vi "MAIN - Template Application.vi"() -> ()   [LabVIEW 2012, in "Car Wash.lvlib"]
uses:
  Car Wash.lvlib
  Components/State Declaration.ctl
  Components/System Trigger.ctl
  Components/System Trigger Element.ctl
  <vilib>/Utility/error.llb/DialogTypeEnum.ctl
  Components/AMC/Read Termination Message.vi
  Components/AMC/Update Message Routing Info.vi
  Components/AMC/Create Multiple Messages.vi
  Components/AMC/Create Single Message.vi
  Components/TypeDef - SHIFTER.ctl
  Components/AMC/Globals.vi
  Components/AMC/Send Message.vi
  Components/Dependencies.llb/TLB`_Dependencies.lvlib
  Components/AMC/AMC.lvlib
panel:
  out "Status":string
  in  "Start Wash":bool
  in  "Reset Car":bool
  out "Wash Progress":dbl(slide) scale=0.0..6.0
  in  "Giant Blowdryers":bool
  in  "Rinse":bool
  in  "Wax":bool
  in  "Roller Brushes":bool
  in  "Soap":bool
  in  "Pre-Soak":bool
  out "error out":errorcluster
  # "Car Wash"
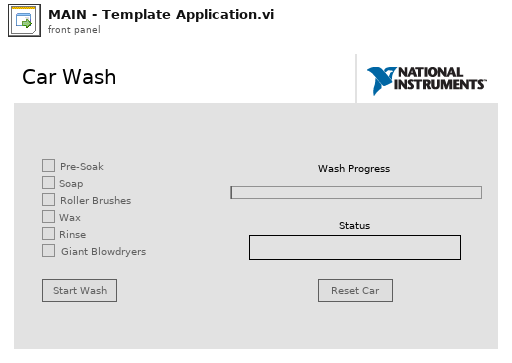
[diagram p1: front panel]
types:
  T1 = typedef "Car Wash.lvlib/System Trigger.ctl" = enum16{"<None>", "Cache User Parameters", "Close Application", "Start Wash", "Reset Car"}
  T2 = typedef "Car Wash.lvlib/State Declaration.ctl" = enum16{"<Startup>", "Idle", "Washing", "Done Washing", "<Shutdown>"}
  T3 = enum16{"Clear SR", "Set Display", "Set Shifter", "Initialize Events", "Init Q"}
  T4 = typedef "Car Wash.lvlib/TypeDef - SHIFTER.ctl" = cluster{"State":T2, "User Data":cluster{"Active Item Tag":string, "Pre-Soak":bool, "Soap":bool, "Roller Brushes":bool, "Wax":bool, "Rinse":bool, "Giant Blowdryers":bool}, "Display Data":cluster{"Active Item Tag":string, "Wash Progress":dbl, "Status":string}, "User Parameter Controls":refnum<vi>[], "Framework Data":cluster{"Exit Event":T5, "Terminate Error":errorcluster}, "Private Data":cluster{"Active Item Tag":string, "Step Booleans Array":bool[], "Step Names Array":string[]}}
  T5 = typedef "Car Wash.lvlib/TLB`_Dependencies.lvlib/Exit Event Ref.ctl" = refnum<user-event>
  T6 = typedef "Car Wash.lvlib/System Trigger Element.ctl" = cluster{"System Triggers":T1, "Trigger Data":variant}
  T7 = typedef "Car Wash.lvlib/AMC.lvlib/Message Queue.ctl" = refnum<queue>
  T8 = enum8{"Enabled", "Disabled", "Disabled and Grayed Out"}
  T9 = typedef "DialogTypeEnum.ctl" = enum16{"no dialog", "OK message", "continue or stop message", "auto error handling dialog", "OK message + warnings", "continue/stop + warnings"}
  T10 = enum32{"Invalid", "Standard", "Closed", "Hidden", "Minimized", "Maximized"}
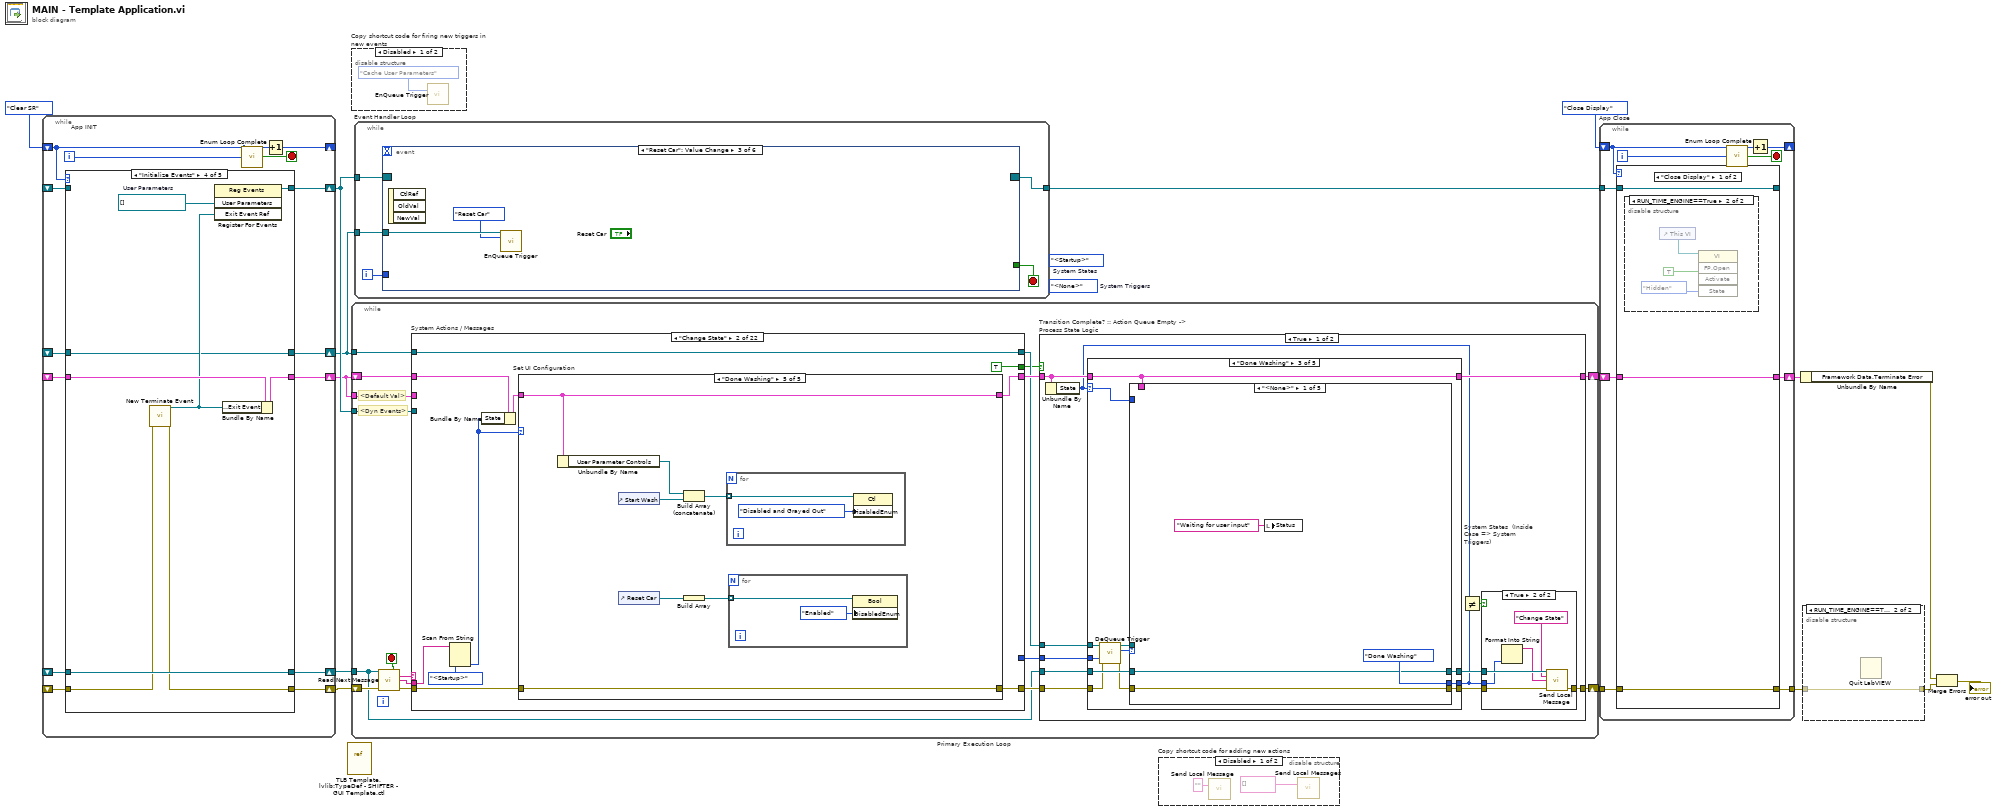
[diagram p0: block diagram]
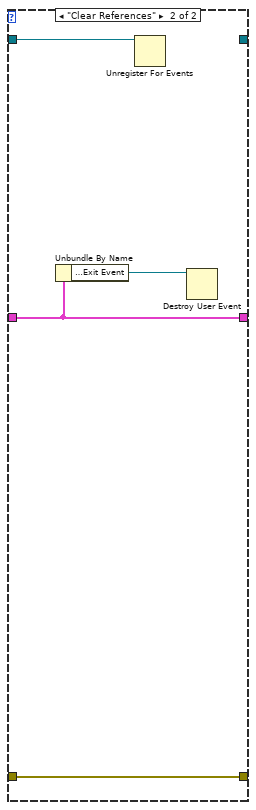
[diagram p6: hidden frame]
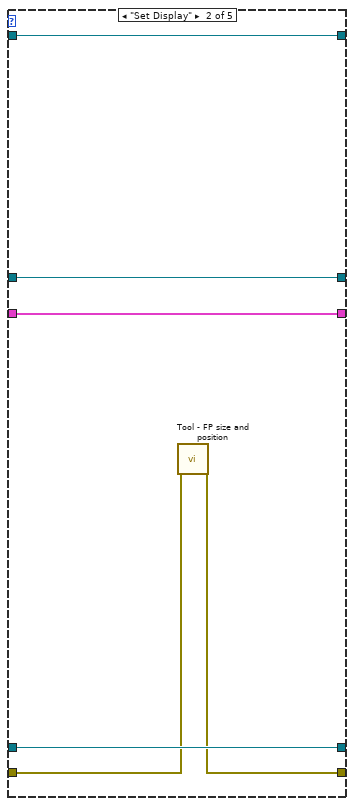
[diagram p8: hidden frame]
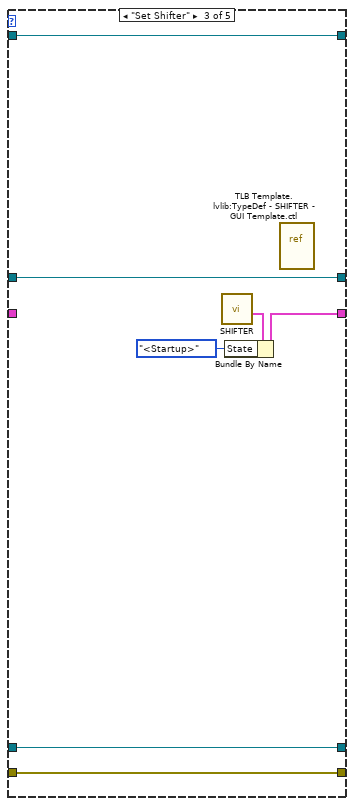
[diagram p9: hidden frame]
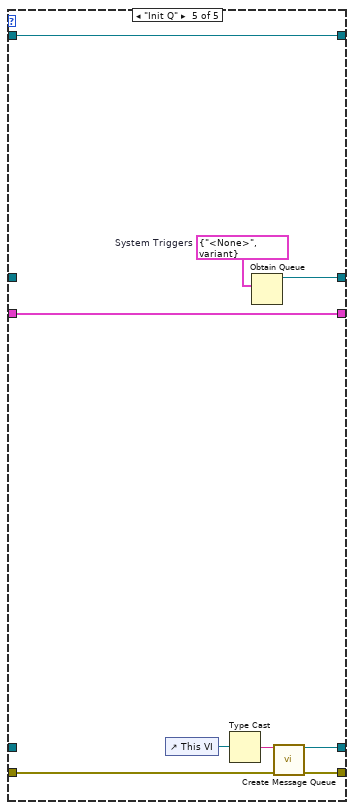
[diagram p10: hidden frame]
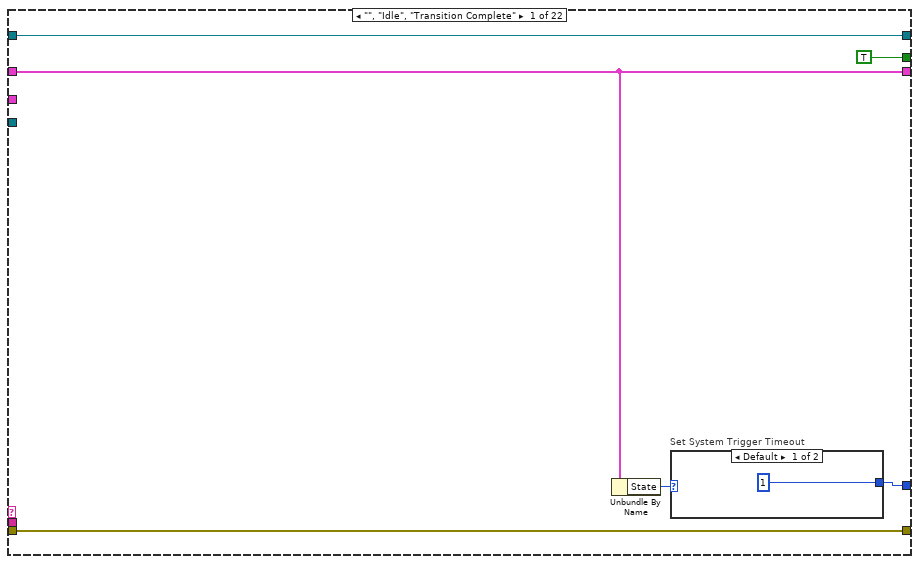
[diagram p11: hidden frame]
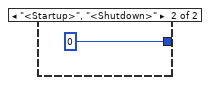
[diagram p12: hidden frame]
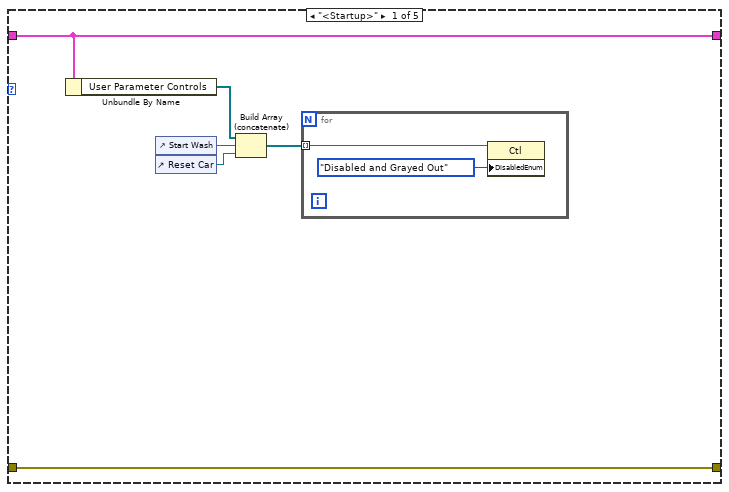
[diagram p13: hidden frame]
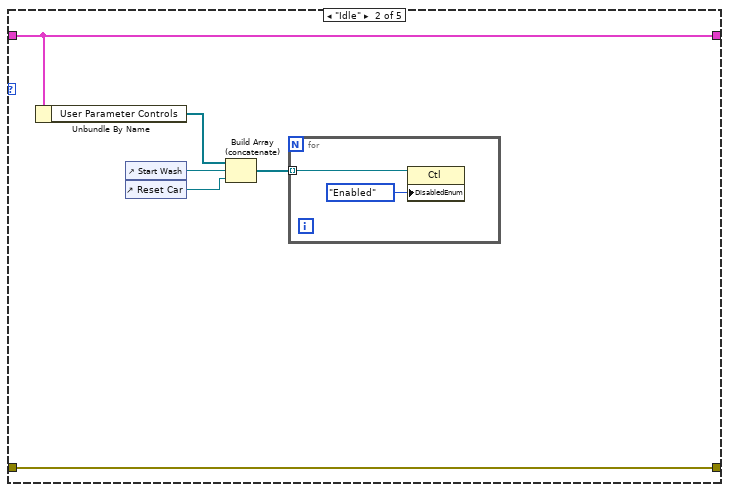
[diagram p14: hidden frame]
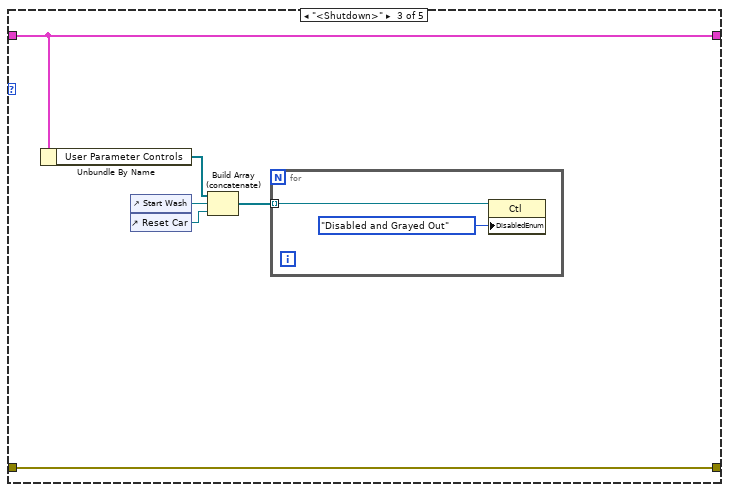
[diagram p15: hidden frame]
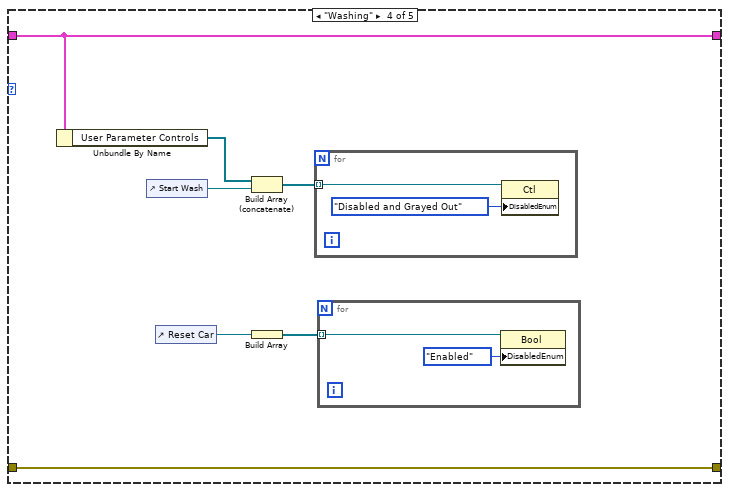
[diagram p16: hidden frame]
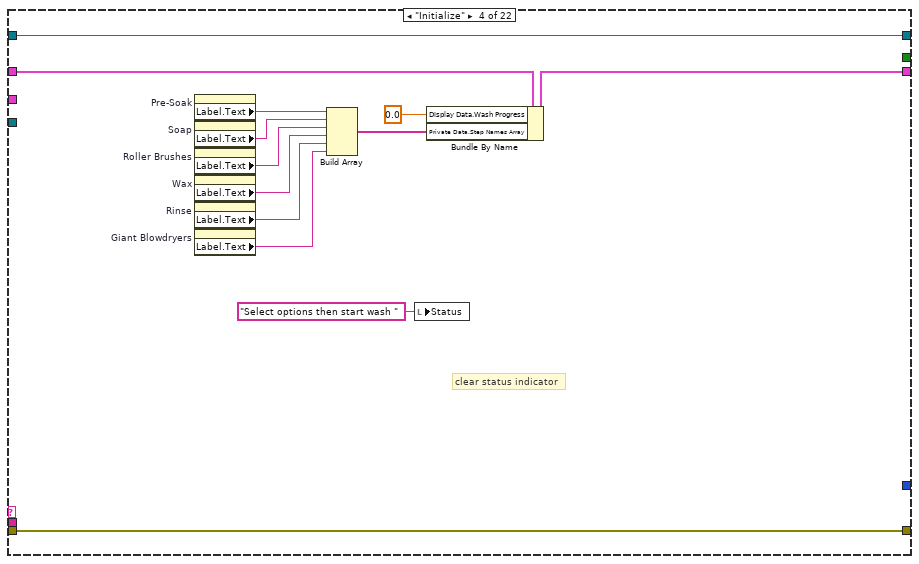
[diagram p18: hidden frame]
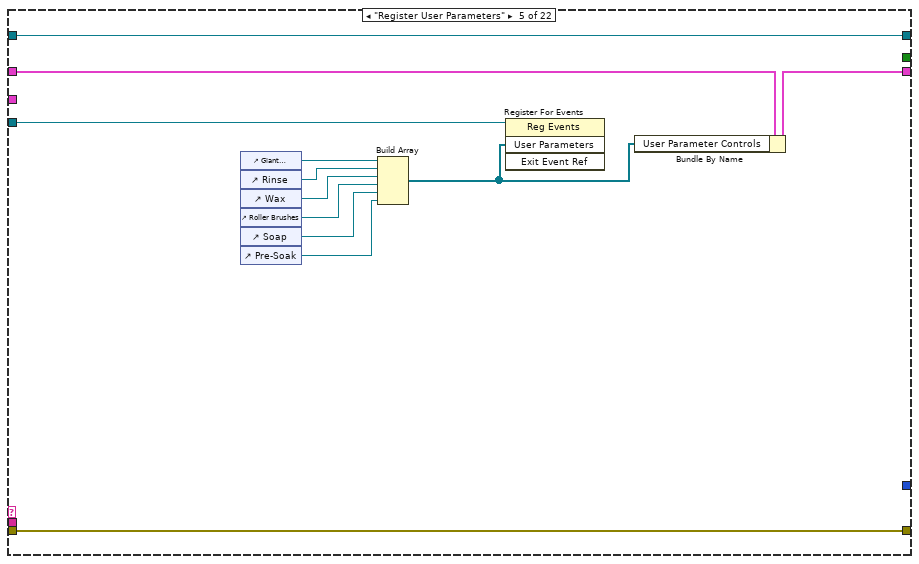
[diagram p19: hidden frame]
diagram:
  (unwired) System_Trigger."<None>"  # System Triggers
  (unwired) State_Declaration."<Startup>"  # System States
  n1 = while "App INIT" {
    shift-right: [w23] -> _
    shift-left: T3."Clear SR" -> [w18]
    shift-right: [w29] -> w9
    shift-left: _ -> [w22]
    shift-right: [w26] -> w8
    shift-left: _ -> [w21]
    shift-right: [w28] -> w11
    shift-left: _ -> [w20]
    shift-right: [w27] -> w1
    shift-left: _ -> [w19]
    shift-right: [w17] -> w2
    shift-left: _ -> [w16]
    i -> [w24]
    stop <- w25 stop-if-true
    n2 = case shown="\"Initialize Events\"" w18 {
      tunnel: [_ w33 w42 w51 w56] -> w29
      tunnel: [_ w31 w41 w44 w55] -> w26
      tunnel: [_ w35 w36 w48 w54] -> w27
      tunnel: [_ w34 w40 w47 w60] -> w28
      tunnel: w22 -> [_ w33 w42 w51 _]
      tunnel: w21 -> [_ w32 w41 w45 w59]
      tunnel: w20 -> [_ w34 w40 _ w60]
      tunnel: w19 -> [_ w35 _ w49 w54]
      tunnel: [_ w30 w39 w43 w58] -> w17
      tunnel: w16 -> [_ w30 w39 w43 _]
      frame "Clear SR" {
      }
      frame "Set Display" {
        n3 = call "Tool - FP size and position.vi"("error in (no error)"=w32) -> ("error out"=w31:errorcluster)  [unwired: 7 in, 11 out]
      }
      frame "Set Shifter" {
        n4 = call "SHIFTER.vi"() -> ("SHIFTER DATA"=w37:T4)  [unwired: 15 in]
        n5 = Bundle By Name(cluster=w37, "State"=State_Declaration."<Startup>") -> (w36:T4)
        n6 = vi-ref "TLB Template.lvlib:TypeDef - SHIFTER - GUI Template.ctl"() -> ()  [unwired: 1 out]
      }
      frame "Initialize Events" {
        w50 = refnum<vi>[] []  # User Parameters
        n7 = call "New Terminate Event.vi"("error in (no error)"=w45) -> ("Exit Event Ref"=w46:T5, "error out"=w44:errorcluster)  [unwired: 13 in]
        n8 = register-events(w50, w46) -> (reference out=w47:refnum<event-registration>)  [unwired: 2 in, 1 out]
        n9 = Bundle By Name(cluster=w49, "Framework Data.Exit Event"=w46) -> (w48:T4)
      }
      frame "Init Q" {
        w57 = T6 {"System Triggers"=enum."<None>", "Trigger Data"=variant}  # System Triggers
        n10 = control-ref of="This VI"() -> (w53:refnum<vi>)
        n11 = Type Cast(x=w53) -> (*(type *) &x=w52:string)  [unwired: 1 in]
        n12 = Obtain Queue(element data type=w57) -> (queue out=w58:refnum<queue>)  [unwired: 4 in, 2 out]
        n13 = call "Create Message Queue.vi"("message queue name"=w52, "error in"=w59) -> ("message queue out"=w56:T7, "error out"=w55:errorcluster)  [unwired: 12 in]
      }
    }
    n14 = call "Enum Loop Complete.vi"("Current State Enum"=w18, "Itteration"=w24) -> ("Loop Complete?"=w25:bool)  [unwired: 13 out]
    n15 = Increment(x=w18) -> (x+1=w23:T3)
  }
  n16 = vi-ref "TLB Template.lvlib:TypeDef - SHIFTER - GUI Template.ctl"() -> ()  [unwired: 1 out]
  n17 = disable-structure "Copy shortcut code for firing new triggers in new events" shown="Disabled" {
    frame Disabled {
      n18 = call "EnQueue Trigger.vi"("System Triggers"=System_Trigger."Cache User Parameters") -> ()  [unwired: 13 in, 2 out]
    }
    frame Enabled {
    }
  }
  n19 = while "Primary Execution Loop" {
    shift-right: [w68] -> w15
    shift-left: w8 -> [w75]
    shift-right: [w71] -> w14
    shift-left: w1 -> [w78]
    tunnel: w1 -> [w77]
    tunnel: w9 -> [w66]
    tunnel: w11 -> [w76]
    tunnel: w2 -> [w67]
    stop <- w73 stop-if-true
    # "<Dyn Events>"
    # "<Default Val>"
    n20 = call "Read Next Message.vi"("message queue in"=w66, "error in"=w75) -> ("exit process?"=w73:bool, "message name"=w72:string, "message value"=w63:string, "error out"=w74:errorcluster)  [unwired: 6 in, 4 out]
    n21 = case "System Actions / Messages" shown="\"Change State\"" w72 {
      selector: w72 -> [_ _ _ _ _ _ _ _ _ _ _ _ _ _ _ _ _ _ _ _ _ w326]
      tunnel: [w84 w91 w145 w157 w170 w173 w181 w187 w190 w201 w207 w215 w224 w236 w248 w260 w272 w284 w292 w297 w320 w330] -> w69
      tunnel: w74 -> [w84 w90 w145 w157 w170 w173 w181 w187 w190 w201 w207 w215 w224 w236 w248 w260 w272 w284 w292 w298 w319 w331]
      tunnel: w78 -> [w79 w87 w144 w156 w169 w172 w183 w185 w188 w193 w204 w213 w220 w232 w244 w256 w268 w280 w291 w295 w323 w332]
      tunnel: w77 -> [_ _ _ _ _ _ _ _ _ _ _ _ _ _ _ _ _ _ _ _ _ _]
      tunnel: [w79 w89 w144 w155 w168 w172 w182 w185 w188 w192 w203 w213 w219 w231 w243 w255 w267 w279 w291 w296 w323 w332] -> w70
      tunnel: [w80 _ _ _ _ _ _ _ _ _ _ _ _ _ _ _ _ _ _ _ _ _] -> w62
      tunnel: w76 -> [_ _ _ _ w167 _ _ _ _ _ _ _ _ _ _ _ _ _ _ _ _ _]
      tunnel: [w82 w95 w143 w158 w166 w171 w180 w186 w189 w200 w206 w214 w223 w235 w247 w259 w271 w283 w290 w293 w317 w324] -> w65
      tunnel: w67 -> [w82 w95 w143 w158 w166 w171 w180 w186 w189 w200 w206 w214 w223 w235 w247 w259 w271 w283 w290 w293 w317 w324]
      tunnel: [TRUE TRUE _ _ _ _ _ _ _ _ _ _ _ _ _ _ _ _ _ _ _ _] -> w64
      tunnel: w63 -> [_ w94 _ _ _ _ _ _ _ _ _ _ _ _ _ _ _ _ _ _ _ _]
      frame "", "Idle", "Transition Complete" {
        n22 = Unbundle By Name(w79) -> ("State"=w81:T2)
        n23 = case "Set System Trigger Timeout" shown="Default" w81 {
          tunnel: [1 0] -> w80
          frame Default {
          }
          frame "<Startup>", "<Shutdown>" {
          }
        }
      }
      frame "Change State" {
        n24 = Scan From String(input string=w94, default 1=State_Declaration."<Startup>" ("State")) -> (output 1=w92:T2)  [unwired: 3 in, 3 out]
        n25 = Bundle By Name(cluster=w87, "State"=w92) -> (w88:T4)
        n26 = case "Set UI Configuration" shown="\"Done Washing\"" w92 {
          tunnel: [w102 w110 w118 w127 w138] -> w91
          tunnel: w90 -> [w102 w110 w118 w127 w138]
          tunnel: [w98 w106 w114 w122 w133] -> w89
          tunnel: w88 -> [w98 w106 w114 w122 w133]
          frame "<Startup>" {
            n27 = Unbundle By Name(w98) -> ("User Parameter Controls"=w97:refnum<vi>[])
            n28 = control-ref of="Start Wash"() -> (w101:refnum<vi>)
            n29 = control-ref of="Reset Car"() -> (w99:refnum<vi>)
            n30 = Build Array (concatenate)(w97, w101, w99) -> (w100:refnum<vi>[])
            n31 = for {
              tunnel: w100 -> [w104] mode=indexing
              n32 = property class="Ctl"(reference=w104, "DisabledEnum"=T8."Disabled and Grayed Out" ("Disabled")) -> ()  [unwired: 1 in, 2 out]
            }
          }
          frame "Idle" {
            n33 = Unbundle By Name(w106) -> ("User Parameter Controls"=w105:refnum<vi>[])
            n34 = control-ref of="Start Wash"() -> (w108:refnum<vi>)
            n35 = control-ref of="Reset Car"() -> (w107:refnum<vi>)
            n36 = Build Array (concatenate)(w105, w108, w107) -> (w109:refnum<vi>[])
            n37 = for {
              tunnel: w109 -> [w112] mode=indexing
              n38 = property class="Ctl"(reference=w112, "DisabledEnum"=T8."Enabled" ("Disabled")) -> ()  [unwired: 1 in, 2 out]
            }
          }
          frame "<Shutdown>" {
            n39 = Unbundle By Name(w114) -> ("User Parameter Controls"=w113:refnum<vi>[])
            n40 = control-ref of="Start Wash"() -> (w116:refnum<vi>)
            n41 = control-ref of="Reset Car"() -> (w115:refnum<vi>)
            n42 = Build Array (concatenate)(w113, w116, w115) -> (w117:refnum<vi>[])
            n43 = for {
              tunnel: w117 -> [w120] mode=indexing
              n44 = property class="Ctl"(reference=w120, "DisabledEnum"=T8."Disabled and Grayed Out" ("Disabled")) -> ()  [unwired: 1 in, 2 out]
            }
          }
          frame "Washing" {
            n45 = Unbundle By Name(w122) -> ("User Parameter Controls"=w121:refnum<vi>[])
            n46 = control-ref of="Start Wash"() -> (w125:refnum<vi>)
            n47 = control-ref of="Reset Car"() -> (w123:refnum<vi>)
            n48 = Build Array (concatenate)(w121, w125) -> (w126:refnum<vi>[])
            n49 = Build Array(w123) -> (w124:refnum<vi>[])
            n50 = for {
              tunnel: w126 -> [w131] mode=indexing
              n51 = property class="Ctl"(reference=w131, "DisabledEnum"=T8."Disabled and Grayed Out" ("Disabled")) -> ()  [unwired: 1 in, 2 out]
            }
            n52 = for {
              tunnel: w124 -> [w129] mode=indexing
              n53 = property class="Bool"(reference=w129, "DisabledEnum"=T8."Enabled" ("Disabled")) -> ()  [unwired: 1 in, 2 out]
            }
          }
          frame "Done Washing" {
            n54 = Unbundle By Name(w133) -> ("User Parameter Controls"=w132:refnum<vi>[])
            n55 = control-ref of="Start Wash"() -> (w136:refnum<vi>)
            n56 = control-ref of="Reset Car"() -> (w134:refnum<vi>)
            n57 = Build Array (concatenate)(w132, w136) -> (w137:refnum<vi>[])
            n58 = Build Array(w134) -> (w135:refnum<vi>[])
            n59 = for {
              tunnel: w137 -> [w142] mode=indexing
              n60 = property class="Ctl"(reference=w142, "DisabledEnum"=T8."Disabled and Grayed Out" ("Disabled")) -> ()  [unwired: 1 in, 2 out]
            }
            n61 = for {
              tunnel: w135 -> [w140] mode=indexing
              n62 = property class="Bool"(reference=w140, "DisabledEnum"=T8."Enabled" ("Disabled")) -> ()  [unwired: 1 in, 2 out]
            }
          }
        }
      }
      frame "/*********Initialize********/" {
      }
      frame "Initialize" {
        # "clear status indicator"
        n63 = property on="Pre-Soak" class="Bool (strict)"() -> ("Label.Text"=w152:string)  [unwired: 2 in, 2 out]
        n64 = property on="Soap" class="Bool (strict)"() -> ("Label.Text"=w151:string)  [unwired: 2 in, 2 out]
        n65 = property on="Roller Brushes" class="Bool (strict)"() -> ("Label.Text"=w150:string)  [unwired: 2 in, 2 out]
        n66 = property on="Wax" class="Bool (strict)"() -> ("Label.Text"=w149:string)  [unwired: 2 in, 2 out]
        n67 = property on="Rinse" class="Bool (strict)"() -> ("Label.Text"=w148:string)  [unwired: 2 in, 2 out]
        n68 = property on="Giant Blowdryers" class="Bool (strict)"() -> ("Label.Text"=w147:string)  [unwired: 2 in, 2 out]
        n69 = Build Array(w152, w151, w150, w149, w148, w147) -> (w146:string[])
        n70 = local write "Status"("Select options then start wash " ("Status")) -> ()
        n71 = Bundle By Name(cluster=w156, "Display Data.Wash Progress"=0.0, "Private Data.Step Names Array"=w146) -> (w155:T4)
      }
      frame "Register User Parameters" {
        n72 = control-ref of="Giant Blowdryers"() -> (w165:refnum<vi>)
        n73 = control-ref of="Rinse"() -> (w160:refnum<vi>)
        n74 = control-ref of="Wax"() -> (w161:refnum<vi>)
        n75 = control-ref of="Roller Brushes"() -> (w162:refnum<vi>)
        n76 = control-ref of="Soap"() -> (w163:refnum<vi>)
        n77 = control-ref of="Pre-Soak"() -> (w164:refnum<vi>)
        n78 = Build Array(w165, w160, w161, w162, w163, w164) -> (w159:refnum<vi>[])
        n79 = register-events(reference=w167, w159) -> ()  [unwired: 2 in, 2 out]
        n80 = Bundle By Name(cluster=w169, "User Parameter Controls"=w159) -> (w168:T4)
      }
      frame "/*********Display Updates********/" {
      }
      frame "Cache User Parameters" {
        n81 = Bundle By Name(cluster=w183, "User Data.Pre-Soak"="Pre-Soak", "User Data.Soap"="Soap", "User Data.Roller Brushes"="Roller Brushes", "User Data.Wax"="Wax", "User Data.Rinse"="Rinse", "User Data.Giant Blowdryers"="Giant Blowdryers") -> (w182:T4)
      }
      frame "Update Display" {
        # "status updated via local variable"
        n82 = Unbundle By Name(w185) -> ("Display Data.Wash Progress"=→"Wash Progress":dbl)
      }
      frame "/*********Primary Execution********/" {
      }
      frame "Create Steps Array" {
        n83 = Unbundle By Name(w193) -> ("User Data.Pre-Soak"=w199:bool, "User Data.Soap"=w198:bool, "User Data.Roller Brushes"=w197:bool, "User Data.Wax"=w196:bool, "User Data.Rinse"=w195:bool, "User Data.Giant Blowdryers"=w194:bool)
        n84 = Build Array(w199, w198, w197, w196, w195, w194) -> (w191:bool[])
        n85 = Bundle By Name(cluster=w193, "Private Data.Step Booleans Array"=w191) -> (w192:T4)
      }
      frame "Increment Step" {
        n86 = Unbundle By Name(w204) -> ("Display Data.Wash Progress"=w205:dbl)
        n87 = Increment(x=w205) -> (x+1=w202:dbl)
        n88 = Bundle By Name(cluster=w204, "Display Data.Wash Progress"=w202) -> (w203:T4)
      }
      frame "Evaluate Step" {
        n89 = Unbundle By Name(w213) -> ("Display Data.Wash Progress"=w210:dbl, "Private Data.Step Booleans Array"=w212:bool[], "Private Data.Step Names Array"=w211:string[])
        n90 = Index Array(array=w211, index=w210) -> (element=w208:string)
        n91 = Index Array(array=w212, index=w210) -> (element=w209:bool)
        n92 = case shown="True" w209 {
          tunnel: w208 -> [_ w217]
          frame False {
          }
          frame True {
            n93 = local write "Status"(w217) -> ()
            n94 = Wait (ms)(milliseconds to wait=u32 1000 ("millisecond timer value")) -> ()  [unwired: 1 out]
          }
        }
      }
      frame "Pre-Soak" {
        n95 = Unbundle By Name(w220) -> ("Display Data.Wash Progress"=w222:dbl)
        n96 = Unbundle By Name(w220) -> ("User Data.Pre-Soak"=w218:bool)
        n97 = case shown="True" w218 {
          tunnel: w222 -> [w225 w229]
          tunnel: [w225 w228] -> w221
          frame False {
          }
          frame True {
            n98 = Increment(x=w229) -> (x+1=w228:dbl)
            n99 = local write "Status"("Pre-Soak" ("Status")) -> ()
            n100 = Wait (ms)(milliseconds to wait=u32 1000) -> ()  [unwired: 1 out]
          }
        }
        n101 = Bundle By Name(cluster=w220, "Display Data.Wash Progress"=w221) -> (w219:T4)
      }
      frame "Soap" {
        n102 = Unbundle By Name(w232) -> ("Display Data.Wash Progress"=w234:dbl)
        n103 = Unbundle By Name(w232) -> ("User Data.Soap"=w230:bool)
        n104 = case shown="True" w230 {
          tunnel: w234 -> [w237 w241]
          tunnel: [w237 w240] -> w233
          frame False {
          }
          frame True {
            n105 = Increment(x=w241) -> (x+1=w240:dbl)
            n106 = local write "Status"("Soap" ("Status")) -> ()
            n107 = Wait (ms)(milliseconds to wait=u32 1000) -> ()  [unwired: 1 out]
          }
        }
        n108 = Bundle By Name(cluster=w232, "Display Data.Wash Progress"=w233) -> (w231:T4)
      }
      frame "Roller Brushes" {
        n109 = Unbundle By Name(w244) -> ("Display Data.Wash Progress"=w246:dbl)
        n110 = Unbundle By Name(w244) -> ("User Data.Roller Brushes"=w242:bool)
        n111 = case shown="True" w242 {
          tunnel: w246 -> [w249 w253]
          tunnel: [w249 w252] -> w245
          frame False {
          }
          frame True {
            n112 = Increment(x=w253) -> (x+1=w252:dbl)
            n113 = local write "Status"("Roller Brushes" ("Status")) -> ()
            n114 = Wait (ms)(milliseconds to wait=u32 1000) -> ()  [unwired: 1 out]
          }
        }
        n115 = Bundle By Name(cluster=w244, "Display Data.Wash Progress"=w245) -> (w243:T4)
      }
      frame "Wax" {
        n116 = Unbundle By Name(w256) -> ("Display Data.Wash Progress"=w258:dbl)
        n117 = Unbundle By Name(w256) -> ("User Data.Wax"=w254:bool)
        n118 = case shown="True" w254 {
          tunnel: w258 -> [w261 w265]
          tunnel: [w261 w264] -> w257
          frame False {
          }
          frame True {
            n119 = Increment(x=w265) -> (x+1=w264:dbl)
            n120 = local write "Status"("Wax" ("Status")) -> ()
            n121 = Wait (ms)(milliseconds to wait=u32 1000) -> ()  [unwired: 1 out]
          }
        }
        n122 = Bundle By Name(cluster=w256, "Display Data.Wash Progress"=w257) -> (w255:T4)
      }
      frame "Rinse" {
        n123 = Unbundle By Name(w268) -> ("Display Data.Wash Progress"=w270:dbl)
        n124 = Unbundle By Name(w268) -> ("User Data.Rinse"=w266:bool)
        n125 = case shown="True" w266 {
          tunnel: w270 -> [w273 w277]
          tunnel: [w273 w276] -> w269
          frame False {
          }
          frame True {
            n126 = Increment(x=w277) -> (x+1=w276:dbl)
            n127 = local write "Status"("Rinse" ("Status")) -> ()
            n128 = Wait (ms)(milliseconds to wait=u32 1000) -> ()  [unwired: 1 out]
          }
        }
        n129 = Bundle By Name(cluster=w268, "Display Data.Wash Progress"=w269) -> (w267:T4)
      }
      frame "Giant Blowdryers" {
        n130 = Unbundle By Name(w280) -> ("Display Data.Wash Progress"=w282:dbl)
        n131 = Unbundle By Name(w280) -> ("User Data.Giant Blowdryers"=w278:bool)
        n132 = case shown="True" w278 {
          tunnel: w282 -> [w285 w289]
          tunnel: [w285 w288] -> w281
          frame False {
          }
          frame True {
            n133 = Increment(x=w289) -> (x+1=w288:dbl)
            n134 = local write "Status"("Giant Blowdryers" ("Status")) -> ()
            n135 = Wait (ms)(milliseconds to wait=u32 1000) -> ()  [unwired: 1 out]
          }
        }
        n136 = Bundle By Name(cluster=w280, "Display Data.Wash Progress"=w281) -> (w279:T4)
      }
      frame "/*********Shutdown********/" {
      }
      frame "Error" {
        n137 = Unbundle By Name(w295) -> ("State"=w294:T2)
        n138 = case shown="Default" w294 {
          tunnel: w298 -> [w306]
          tunnel: [w305] -> w297
          tunnel: w295 -> [w302]
          tunnel: [w301] -> w296
          tunnel: w293 -> [w299]
          frame Default {
            n139 = call <vilib>:"General Error Handler CORE.vi"("type of dialog (OK msg:1)"=DialogTypeEnum."auto error handling dialog", "error in (no error)"=w306) -> ("stop event propagated"=w304:bool, "error out"=w300:errorcluster)  [unwired: 12 out]
            n140 = case "User Chose to Stop and Not Continue\nFALSE = Continue: CLEAR ERRORS" shown="False" w304 {
              tunnel: [w307 w312] -> w305
              tunnel: w300 -> [w308 w314]
              tunnel: w302 -> [w309 w316]
              tunnel: [w309 w315] -> w301
              tunnel: w299 -> [_ w313]
              frame False {
                n141 = call <vilib>:"Clear Errors.vi"("error in (no error)"=w308) -> ("error out"=w307:errorcluster)  [unwired: 6 out]
              }
              frame True {
                n142 = call <vilib>:"Clear Errors.vi"("error in (no error)"=w314) -> ("error out"=w311:errorcluster)  [unwired: 6 out]
                n143 = Bundle By Name(cluster=w316, "Framework Data.Terminate Error"=w314) -> (w315:T4)
                n144 = call "EnQueue Trigger.vi"("Queue in"=w313, "System Triggers"=System_Trigger."Close Application", "error in (no error)"=w311) -> ("error out"=w312:errorcluster)  [unwired: 11 in, 1 out]
              }
            }
          }
        }
      }
      frame "Exit" {
        w318 = refnum<class> refnum  # event data
        # "Don't wire 'Error In'\nMust Execute Regardless"
        n145 = Unbundle By Name(w323) -> ("Framework Data.Exit Event"=w322:T5)  [unwired: 1 out]
        n146 = Generate User Event(user event=w322, event data cluster=w318) -> (error out=w321:errorcluster)  [unwired: 1 in, 1 out]
        n147 = Merge Errors(w321, w319) -> (w320:errorcluster)
      }
      frame Default {
        w328 = 1 items=["No error", "Argument error", "Memory is full", "Out of zone", "End of file", "File already open", "Generic file I/O error", "File not found", "File permission error", "Disk is full", "Duplicate path", "Too many files open", "System feature not enabled", "Resource file not found", "Cannot add resource", "Resource not found", "Image not found", "Image memory error", "Pen does not exist", "Config type invalid", "Config token not found", "Config parse error", "Config memory error", "Bad external code format", "Bad external code offset", "External code not present", "Null window", "Destroy window error", "Null menu", "Print aborted", "Bad print record", "Print driver error", "Windows error during printing", "Memory error during printing", "Print dialog error", "Generic print error", "Invalid device refnum", "Device not found", "Device parameter error", "Device unit error", "Cannot open device", "Device call aborted", "Generic error", "Cancelled by user", "Object ID too low", "Object ID too high", "Object not in heap", "Unknown heap", "Unknown object (invalid DefProc)", "Unknown object (DefProc not in table)", "Message out of range", "Invalid (null) method", "Unknown message", "Manager call not supported", "Bad address", "Network operation in progress", "Network operation timed out", "Connection is busy", "Network attribute not supported", "Network error", "Address in use", "System out of memory", "Connection aborted", "Connection refused", "Not connected", "Already connected", "Connection closed", "Initialization error (interapplication manager)", "Bad occurrence", "Wait on unbound occurrence handler", "Occurrence queue overflow", "Datalog type conflict", "Unused", "Unrecognized type (interapplication manager)", "Memory corrupt", "Failed to make temporary DLL", "Old CIN version", "Drag socket not found", "Failed to load drop-object", "Failed to register OLE object", "Failed to release OLE object", "Format specifier type mismatch", "Unknown format specifier", "Too few format specifiers", "Too many format specifiers", "Scan failed", "Newer CIN version", "Error converting to variant", "Runtime menu error", "Password tampered", "Variant attribute not found", "Incompatible variant data type", "Event data is not available", "Event Store is not present", "Occurrence is not found", "Event Queue is not created", "Event info is not available", "Refnum passed is NULL", "Error retrieving Class GUID", "Error retrieving CoClass GUID", "Error retrieving TypeLib GUID.", "Bad built application magic bytes.", "Specific driver is different from the specific driver associated with the Logical Name.", "There is no session opened to the class driver.", "Max Error", "MAX - Error with config objects", "MAX - Error loading configuration", "MAX - Group not supported"]
        w329 = TRUE  # status
        n148 = Format Into String(format string="DEVELOPER ERROR:\nImproper Action Requested\n================\nAction {%s} does not exist within this architecture\n\nCheck for spelling and case errors" ("source"), w326) -> (resulting string=w327:string)  [unwired: 2 in, 1 out]
        n149 = Bundle By Name(cluster=w331, "status"=w329, "code"=w328, "source"=w327) -> (w330:errorcluster)
      }
    }
    n150 = case "Transition Complete? :: Action Queue Empty -> Process State Logic" shown="True" w64 {
      tunnel: [w344 w497] -> w71
      tunnel: w70 -> [w334 w497]
      tunnel: w69 -> [w343 w496]
      tunnel: w66 -> [w342 _]
      tunnel: [w338 w496] -> w68
      tunnel: w65 -> [w341 _]
      tunnel: w62 -> [w335 _]
      frame True {
        n151 = Unbundle By Name(w334) -> ("State"=w333:T2)
        n152 = case "System States  (Inside Case => System Triggers)" shown="\"Done Washing\"" w333 {
          selector: w333 -> [_ w373 w406 w440 _]
          tunnel: [w360 w379 w412 w446 w487] -> w344
          tunnel: w334 -> [w360 w379 w412 w446 w487]
          tunnel: w343 -> [w354 w371 w404 w438 w481]
          tunnel: w342 -> [w352 w375 w408 w442 w479]
          tunnel: [w359 w378 w411 w445 w486] -> w339
          tunnel: w341 -> [w362 w380 w413 w447 w489]
          tunnel: [w358 w377 w410 w444 w485] -> w340
          tunnel: [w357 w376 w409 w443 w484] -> w337
          tunnel: w335 -> [w356 w369 w402 w436 w483]
          frame "<Startup>" {
            n153 = call "DeQueue Trigger.vi"("Queue in"=w362, "Timeout (0)"=w356, "error in (no error)"=w354) -> ("Queue out"=w355:refnum<queue>, "System Triggers"=w361:T1, "error out"=w353:errorcluster)  [unwired: 9 in, 1 out]
            n154 = case shown="\"<None>\", Default" w361 {
              tunnel: w360 -> [_]
              tunnel: [w366] -> w359
              tunnel: w353 -> [w367]
              tunnel: w352 -> [w365]
              tunnel: [w364] -> w358
              tunnel: [State_Declaration."Idle" ("State")] -> w357
              tunnel: w355 -> [_]
              frame "<None>", Default {
                w363 = string[] ["Initialize", "Cache User Parameters", "Register User Parameters", "Update Display"]  # Initial Elements
                n155 = call "Send Local Messages.vi"("message queue in"=w365, "message names"=w363, "error in"=w367) -> ("message queue out"=w364:T7, "error out"=w366:errorcluster)  [unwired: 10 in, 1 out]
              }
            }
          }
          frame "Idle" {
            n156 = call "DeQueue Trigger.vi"("Queue in"=w380, "Timeout (0)"=w369, "error in (no error)"=w371) -> ("Queue out"=w374:refnum<queue>, "System Triggers"=w372:T1, "error out"=w370:errorcluster)  [unwired: 9 in, 1 out]
            n157 = case shown="\"Start Wash\"" w372 {
              tunnel: w379 -> [_ _ _ _ _]
              tunnel: [w381 w385 w389 w394 w398] -> w378
              tunnel: w370 -> [w381 w385 w392 w394 w399]
              tunnel: w375 -> [w382 w386 w391 w395 w396]
              tunnel: [w382 w386 w390 w395 w397] -> w377
              tunnel: [State_Declaration."Idle" ("State") State_Declaration."<Shutdown>" ("State") w387 State_Declaration."Idle" ("State") State_Declaration."Washing" ("State")] -> w376
              tunnel: w374 -> [_ _ _ _ _]
              tunnel: w373 -> [_ _ w387 _ _]
              frame "<None>" {
              }
              frame "Close Application" {
              }
              frame "Cache User Parameters" {
                n158 = call "Send Local Message.vi"("message queue in"=w391, "message name"="Cache User Parameters" ("Message Name"), "error in"=w392) -> ("message queue out"=w390:T7, "error out"=w389:errorcluster)  [unwired: 10 in, 1 out]
              }
              frame Default {
              }
              frame "Start Wash" {
                n159 = call "Send Local Messages.vi"("message queue in"=w396, "message names"=string[] ["Create Steps Array"], "error in"=w399) -> ("message queue out"=w397:T7, "error out"=w398:errorcluster)  [unwired: 10 in, 1 out]
              }
            }
          }
          frame "Done Washing" {
            n160 = call "DeQueue Trigger.vi"("Queue in"=w413, "Timeout (0)"=w402, "error in (no error)"=w404) -> ("Queue out"=w407:refnum<queue>, "System Triggers"=w405:T1, "error out"=w403:errorcluster)  [unwired: 9 in, 1 out]
            n161 = case shown="\"<None>\"" w405 {
              tunnel: w412 -> [_ _ _ _ _]
              tunnel: [w415 w419 w424 w429 w434] -> w411
              tunnel: w403 -> [w415 w419 w425 w432 w434]
              tunnel: w408 -> [w416 w420 w423 w431 w435]
              tunnel: [w416 w420 w422 w430 w435] -> w410
              tunnel: [State_Declaration."Done Washing" ("State") State_Declaration."<Shutdown>" ("State") State_Declaration."Idle" ("State") w427 State_Declaration."Idle" ("State")] -> w409
              tunnel: w407 -> [_ _ _ _ _]
              tunnel: w406 -> [_ _ _ w427 _]
              frame "<None>" {
                n162 = local write "Status"("Waiting for user input" ("Status")) -> ()
              }
              frame "Close Application" {
              }
              frame "Reset Car" {
                n163 = call "Send Local Messages.vi"("message queue in"=w423, "message names"=string[] ["Initialize", "Update Display"], "error in"=w425) -> ("message queue out"=w422:T7, "error out"=w424:errorcluster)  [unwired: 10 in, 1 out]
              }
              frame "Cache User Parameters" {
                n164 = call "Send Local Message.vi"("message queue in"=w431, "message name"="Cache User Parameters" ("Message Name"), "error in"=w432) -> ("message queue out"=w430:T7, "error out"=w429:errorcluster)  [unwired: 10 in, 1 out]
              }
              frame Default {
              }
            }
          }
          frame "Washing" {
            n165 = call "DeQueue Trigger.vi"("Queue in"=w447, "Timeout (0)"=w436, "error in (no error)"=w438) -> ("Queue out"=w441:refnum<queue>, "System Triggers"=w439:T1, "error out"=w437:errorcluster)  [unwired: 9 in, 1 out]
            n166 = case shown="\"<None>\"" w439 {
              tunnel: w446 -> [w455 _ _ _ _]
              tunnel: [w458 w464 w468 w472 w477] -> w445
              tunnel: w437 -> [w459 w465 w468 w475 w477]
              tunnel: w442 -> [w457 w463 w469 w474 w478]
              tunnel: [w456 w462 w469 w473 w478] -> w444
              tunnel: [w448 State_Declaration."Idle" ("State") State_Declaration."<Shutdown>" ("State") w470 State_Declaration."Idle" ("State")] -> w443
              tunnel: w441 -> [_ _ _ _ _]
              tunnel: w440 -> [_ _ _ w470 _]
              frame "<None>" {
                n167 = Unbundle By Name(w455) -> ("Display Data.Wash Progress"=w453:dbl, "Private Data.Step Booleans Array"=w454:bool[])
                n168 = call "Send Local Messages.vi"("message queue in"=w457, "message names"=string[] ["Evaluate Step", "Increment Step", "Update Display"], "error in"=w459) -> ("message queue out"=w456:T7, "error out"=w458:errorcluster)  [unwired: 10 in, 1 out]
                n169 = Array Size(array=w454) -> (size(s)=w452:i32)
                n170 = Equal?(x=w453, y=w452) -> (x = y?=w451:bool)
                n171 = Select(t=State_Declaration."Done Washing" ("State"), s=w451, f=State_Declaration."Washing" ("State")) -> (s? t:f=w448:T2)
              }
              frame "Reset Car" {
                n172 = call "Send Local Messages.vi"("message queue in"=w463, "message names"=string[] ["Initialize", "Update Display"], "error in"=w465) -> ("message queue out"=w462:T7, "error out"=w464:errorcluster)  [unwired: 10 in, 1 out]
              }
              frame "Close Application" {
              }
              frame "Cache User Parameters" {
                n173 = call "Send Local Message.vi"("message queue in"=w474, "message name"="Cache User Parameters" ("Message Name"), "error in"=w475) -> ("message queue out"=w473:T7, "error out"=w472:errorcluster)  [unwired: 10 in, 1 out]
              }
              frame Default {
              }
            }
          }
          frame "<Shutdown>" {
            n174 = call "DeQueue Trigger.vi"("Queue in"=w489, "Timeout (0)"=w483, "error in (no error)"=w481) -> ("Queue out"=w482:refnum<queue>, "System Triggers"=w488:T1, "error out"=w480:errorcluster)  [unwired: 9 in, 1 out]
            n175 = case shown="\"<None>\", Default" w488 {
              tunnel: w487 -> [_]
              tunnel: [w490] -> w486
              tunnel: w480 -> [w492]
              tunnel: w479 -> [w493]
              tunnel: [w491] -> w485
              tunnel: [State_Declaration."<Shutdown>" ("State")] -> w484
              tunnel: w482 -> [_]
              frame "<None>", Default {
                n176 = call "Send Local Messages.vi"("message queue in"=w493, "message names"=string[] ["Exit"], "error in"=w492) -> ("message queue out"=w491:T7, "error out"=w490:errorcluster)  [unwired: 10 in, 1 out]
              }
            }
          }
        }
        n177 = Not Equal?(x=w333, y=w337) -> (x != y?=w336:bool)
        n178 = case shown="True" w336 {
          tunnel: w340 -> [_ w351]
          tunnel: w339 -> [w345 w350]
          tunnel: [w345 w349] -> w338
          tunnel: w337 -> [_ w347]
          frame False {
          }
          frame True {
            n179 = Format Into String(w347) -> (resulting string=w346:string)  [unwired: 3 in, 1 out]
            n180 = call "Send Local Message.vi"("message queue in"=w351, "message name"="Change State" ("Message Name"), "message value"=w346, "error in"=w350) -> ("error out"=w349:errorcluster)  [unwired: 9 in, 2 out]
          }
        }
      }
      frame False {
      }
    }
  }
  n181 = while "Event Handler Loop" {
    tunnel: w11 -> [w501]
    tunnel: [w500] -> w13
    tunnel: w2 -> [w498]
    i -> [w499]
    stop <- w502 stop-if-true
    n182 = event shown="[2] \"Reset Car\": Value Change" {
      selector: w501 -> [_ _ _ _ _ _]
      dyn-events: [_ _ _ _ _ _] -> w500
      timeout: _ -> [_ _ _ _ _ _]
      tunnel: [_ _ _ _ TRUE ("NewVal") _] -> w502
      tunnel: w499 -> [_ _ _ _ _ _]
      tunnel: w498 -> [w504 w507 w509 _ w520 w524]
      event Panel Close? {
        w505 = TRUE  # Discard?
        n183 = event-data() -> ()  [unwired: 2 out]
        n184 = call "EnQueue Trigger.vi"("Queue in"=w504, "System Triggers"=System_Trigger."Close Application") -> ()  [unwired: 12 in, 2 out]
        n185 = event-data("Discard?"=w505) -> ()  [unwired: 1 in, 1 out]
      }
      event "Start Wash": Value Change {
        n186 = event-data() -> ()  [unwired: 4 out]
        n187 = call "EnQueue Trigger.vi"("Queue in"=w507, "System Triggers"=System_Trigger."Start Wash") -> ()  [unwired: 12 in, 2 out]
      }
      event "Reset Car": Value Change {
        n188 = event-data() -> ()  [unwired: 4 out]
        n189 = call "EnQueue Trigger.vi"("Queue in"=w509, "System Triggers"=System_Trigger."Reset Car") -> ()  [unwired: 12 in, 2 out]
      }
      event Mouse Down {
        n190 = event-data() -> ("Button"=w514:u16, "Mods"=w515:cluster{"Double Click":bool, "Menu Key":bool})  [unwired: 1 out]
        n191 = Unbundle By Name(w515) -> ("Double Click"=w511:bool)
        n192 = Equal?(x=u16 2, y=w514) -> (x = y?=w512:bool)
        n193 = And(x=w512, y=w511) -> (x .and. y?=w510:bool)
        n194 = case "Toggle Menu Visibility :: double RIGHT click on logo" shown="True" w510 {
          frame False {
          }
          frame True {
            n195 = property class="VI"() -> (reference out=w518:refnum<vi>, "TB.Visible"=w516:bool)  [unwired: 2 in, 1 out]
            n196 = Not(x=w516) -> (.not. x?=w517:bool)
            n197 = property class="VI"(reference=w518, "TB.Visible"=w517) -> ()  [unwired: 1 in, 2 out]
          }
        }
      }
      event User Event {
        n198 = event-data() -> ()  [unwired: 2 out]
        n199 = call "EnQueue Trigger.vi"("Queue in"=w520, "System Triggers"=System_Trigger."Close Application") -> ()  [unwired: 12 in, 2 out]
      }
      event Value Change {
        n200 = event-data() -> ()  [unwired: 2 out]
        n201 = call "EnQueue Trigger.vi"("Queue in"=w524, "System Triggers"=System_Trigger."Cache User Parameters") -> ("Queue out"=w523:refnum<queue>)  [unwired: 12 in, 1 out]
        n202 = event "use this event case to register a SPEICIFIC 'User Parameter' for a SPECIFIC action" shown="[0] Timeout" {
          selector: _ -> [_]
          dyn-events: _ -> [_]
          timeout: 0 -> [_]
          tunnel: w523 -> [_]
          event Timeout {
            n203 = event-data() -> ()  [unwired: 1 in, 1 out]
          }
        }
      }
    }
  }
  n204 = disable-structure "Copy shortcut code for adding new actions" shown="Disabled" {
    frame Disabled {
      n205 = call "Send Local Message.vi"("message name"="") -> ()  [unwired: 12 in, 3 out]
      n206 = call "Send Local Messages.vi"("message names"=string[] []) -> ()  [unwired: 12 in, 3 out]
    }
    frame Enabled {
    }
  }
  n207 = while "App Close" {
    shift-right: [w534] -> _
    shift-left: enum16{"Close Display", "Clear References"}."Close Display" -> [w533]
    tunnel: w13 -> [w531]
    tunnel: w15 -> [w532]
    tunnel: [w529] -> w7
    shift-right: [w528] -> w5
    shift-left: w14 -> [w530]
    i -> [w535]
    stop <- w536 stop-if-true
    n208 = case shown="\"Close Display\"" w533 {
      tunnel: [w538 w546] -> w529
      tunnel: [w537 w545] -> w528
      tunnel: [w539 _] -> _
      tunnel: w532 -> [w538 w546]
      tunnel: w531 -> [w539 w543]
      tunnel: w530 -> [w537 w545]
      frame "Close Display" {
        n209 = disable-structure shown="RUN_TIME_ENGINE==True" {
          frame condition #0 (active) {
          }
          frame condition #1 {
            n210 = control-ref of="This VI"() -> (w540:refnum<vi>)
            n211 = invoke class="VI" method="FP.Open"(reference=w540, "Activate"=TRUE ("Activate?"), "State"=T10."Hidden") -> ()  [unwired: 2 in, 5 out]
          }
        }
      }
      frame "Clear References" {
        n212 = Unbundle By Name(w545) -> ("Framework Data.Exit Event"=w544:T5)
        n213 = Unregister For Events(event registration refnum=w543) -> ()  [unwired: 1 in, 1 out]
        n214 = Destroy User Event(user event=w544) -> ()  [unwired: 1 in, 1 out]
      }
    }
    n215 = call "Enum Loop Complete.vi"("Current State Enum"=w533, "Itteration"=w535) -> ("Loop Complete?"=w536:bool)  [unwired: 13 out]
    n216 = Increment(x=w533) -> (x+1=w534:enum16{"Close Display", "Clear References"})
  }
  n217 = Unbundle By Name(w5) -> ("Framework Data.Terminate Error"=w3:errorcluster)
  n218 = disable-structure shown="RUN_TIME_ENGINE==True" {
    disable-tunnel: [w547 w548] -> w4
    disable-tunnel: w7 -> [w547 w548]
    frame condition #0 (active) {
    }
    frame condition #1 {
      n219 = Quit LabVIEW() -> ()  [unwired: 1 in]
    }
  }
  n220 = Merge Errors(w3, w4) -> (→"error out":errorcluster)
